vi "Json_New_Names_Test_Flo.vi"() -> ()   [LabVIEW 2014]
panel:
  out "JSON string":string="{\"label\":\"parms\",\"values\":[{\"chanDescs\":[{\"name\":\"HBCm_U30_01\",\"active\":1},{\"name\":\"HBCm_U30_02\",\"active\":1},{\"name\":\"HBCm_U30_03\",\"active\":1},{\"name\":\"HBCm_U30_04\",\"active\":1},{\"name\":\"HBCm_U30_05\",\"active\":1},{\"name\":\"HBCm_U30_06\",\"active\":1},{\"name\":\"HBCm_U30_07\",\"active\":1},{\"name\":\"HBCm_U30_08\",\"active\":1},{\"name\":\"HBCm_U30_09\",\"active\":1},{\"name\":\"HBCm_U30_10\",\"active\":1},{\"name\":\"HBCm_U30_11\",\"active\":1},{\"name\":\"HBCm_U30_12\",\"active\":1},{\"name\":\"HBCm_U30_13\",\"active\":1},{\"name\":\"HBCm_U30_14\",\"active\":1},{\"name\":\"HBCm_U30_15\",\"active\":1},{\"name\":\"HBCm_U30_16\",\"active\":1},{\"name\":\"HBCm_U30_17\",\"active\":1},{\"name\":\"HBCm_U30_18\",\"active\":1},{\"name\":\"HBCm_U30_19\",\"active\":1},{\"name\":\"HBCm_U30_20\",\"active\":1},{\"name\":\"HBCm_U30_21\",\"active\":1},{\"name\":\"HBCm_U30_22\",\"active\":1},{\"name\":\"HBCm_U30_23\",\"active\":1},{\"name\":\"HBCm_U30_24\",\"active\":1},{\"name\":\"HBCm_U30_25\",\"active\":1},{\"name\":\"HBCm_U30_26\",\"active\":1},{\"name\":\"HBCm_U30_27\",\"active\":1},{\"name\":\"HBCm_U30_28\",\"active\":1},{\"name\":\"HBCm_U30_29\",\"active\":1},{\"name\":\"HBCm_U30_30\",\"active\":1},{\"name\":\"HBCm_U30_31\",\"active\":1},{\"name\":\"HBCm_U30_32\",\"active\":1},{\"name\":\"HBCm_V21_01\",\"active\":1},{\"name\":\"HBCm_V21_02\",\"active\":1},{\"name\":\"HBCm_V21_03\",\"active\":1},{\"name\":\"HBCm_V21_04\",\"active\":1},{\"name\":\"HBCm_V21_05\",\"active\":1},{\"name\":\"HBCm_V21_06\",\"active\":1},{\"name\":\"HBCm_V21_07\",\"active\":1},{\"name\":\"HBCm_V21_08\",\"active\":1},{\"name\":\"HBCm_V21_09\",\"active\":1},{\"name\":\"HBCm_V21_10\",\"active\":1},{\"name\":\"HBCm_V21_11\",\"active\":1},{\"name\":\"HBCm_V21_12\",\"active\":1},{\"name\":\"HBCm_V21_13\",\"active\":1},{\"name\":\"HBCm_V21_14\",\"active\":1},{\"name\":\"HBCm_V21_15\",\"active\":1},{\"name\":\"HBCm_V21_16\",\"active\":1},{\"name\":\"HBCm_V21_17\",\"active\":1},{\"name\":\"HBCm_V21_18\",\"active\":1},{\"name\":\"HBCm_V21_19\",\"active\":1},{\"name\":\"HBCm_V21_20\",\"active\":1},{\"name\":\"HBCm_V21_21\",\"active\":1},{\"name\":\"HBCm_V21_22\",\"active\":1},{\"name\":\"HBCm_V21_23\",\"active\":1},{\"name\":\"HBCm_V21_24\",\"active\":1},{\"name\":\"HBCm_V21_25\",\"active\":1},{\"name\":\"HBCm_V21_26\",\"active\":1},{\"name\":\"HBCm_V21_27\",\"active\":1},{\"name\":\"HBCm_V21_28\",\"active\":1},{\"name\":\"HBCm_V21_29\",\"active\":1},{\"name\":\"HBCm_V21_30\",\"active\":1},{\"name\":\"HBCm_V21_31\",\"active\":1},{\"name\":\"HBCm_V21_32\",\"active\":1},{\"name\":\"HBCm_V21_33\",\"active\":1},{\"name\":\"HBCm_V21_34\",\"active\":1},{\"name\":\"HBCm_V21_35\",\"active\":1},{\"name\":\"HBCm_V21_36\",\"active\":1},{\"name\":\"HBCm_V21_37\",\"active\":1},{\"name\":\"HBCm_V21_38\",\"active\":1},{\"name\":\"HBCm_V21_39\",\"active\":1},{\"name\":\"HBCm_V21_40\",\"active\":1},{\"name\":\"VBCs_V21_01\",\"active\":1},{\"name\":\"VBCs_V21_02\",\"active\":1},{\"name\":\"VBCs_V21_03\",\"active\":1},{\"name\":\"VBCs_V21_04\",\"active\":1},{\"name\":\"VBCs_V21_05\",\"active\":1},{\"name\":\"VBCs_V21_06\",\"active\":1},{\"name\":\"VBCs_V21_08\",\"active\":1},{\"name\":\"VBCs_V21_09\",\"active\":0},{\"name\":\"VBCs_V21_01\",\"active\":1},{\"name\":\"VBCs_V21_02\",\"active\":1},{\"name\":\"VBCs_V21_03\",\"active\":1},{\"name\":\"VBCs_V21_04\",\"active\":1},{\"name\":\"VBCs_V21_05\",\"active\":1},{\"name\":\"VBCs_V21_06\",\"active\":1},{\"name\":\"VBCs_V21_07\",\"active\":1},{\"name\":\"VBCs_V21_08\",\"active\":1},{\"name\":\"VBCs_V21_09\",\"active\":1},{\"name\":\"VBCs_V21_09\",\"active\":1},{\"name\":\"VBCs_V21_10\",\"active\":1},{\"name\":\"VBCs_V21_11\",\"active\":1},{\"name\":\"VBCs_V21_12\",\"active\":1},{\"name\":\"VBCs_V21_13\",\"active\":1},{\"name\":\"VBCs_V21_14\",\"active\":1},{\"name\":\"VBCs_V21_15\",\"active\":1}]}],\"dimensions\":[1399090569999999999,-1]}"
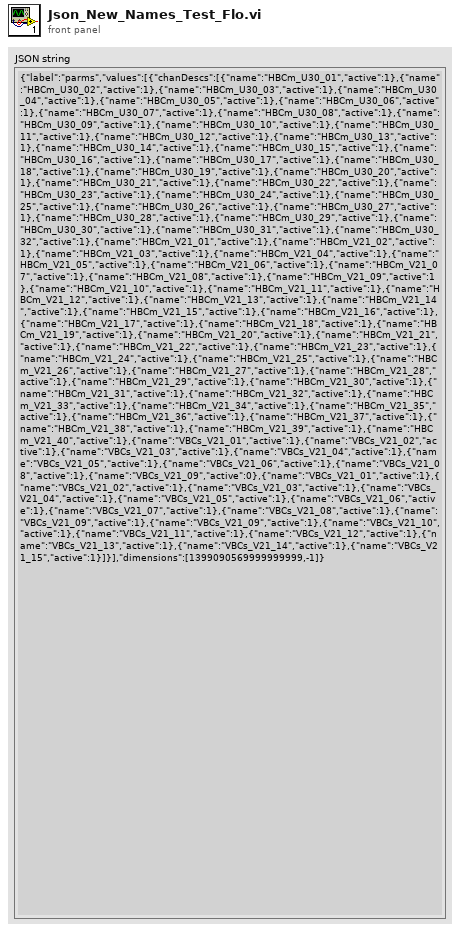
[diagram p1: front panel]
types:
  T1 = cluster{"chanDescs":cluster{"name":string, "active":i32}[]}[]
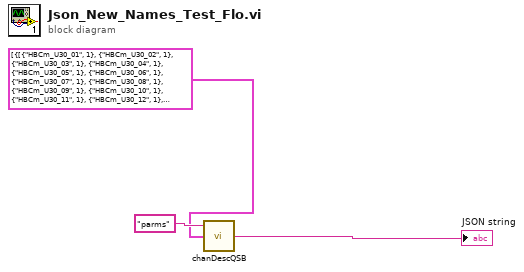
[diagram p0: block diagram]
diagram:
  n1 = call "chanDescQSB.vi"("values"=T1 [{"chanDescs"=[{"name"="HBCm_U30_01", "active"=1}, {"name"="HBCm_U30_02", "active"=1}, {"name"="HBCm_U30_03", "active"=1}, {"name"="HBCm_U30_04", "active"=1}, {"name"="HBCm_U30_05", "active"=1}, {"name"="HBCm_U30_06", "active"=1}, {"name"="HBCm_U30_07", "active"=1}, {"name"="HBCm_U30_08", "active"=1}, {"name"="HBCm_U30_09", "active"=1}, {"name"="HBCm_U30_10", "active"=1}, {"name"="HBCm_U30_11", "active"=1}, {"name"="HBCm_U30_12", "active"=1}, {"name"="HBCm_U30_13", "active"=1}, {"name"="HBCm_U30_14", "active"=1}, {"name"="HBCm_U30_15", "active"=1}, {"name"="HBCm_U30_16", "active"=1}, {"name"="HBCm_U30_17", "active"=1}, {"name"="HBCm_U30_18", "active"=1}, {"name"="HBCm_U30_19", "active"=1}, {"name"="HBCm_U30_20", "active"=1}, {"name"="HBCm_U30_21", "active"=1}, {"name"="HBCm_U30_22", "active"=1}, {"name"="HBCm_U30_23", "active"=1}, {"name"="HBCm_U30_24", "active"=1}, {"name"="HBCm_U30_25", "active"=1}, {"name"="HBCm_U30_26", "active"=1}, {"name"="HBCm_U30_27", "active"=1}, {"name"="HBCm_U30_28", "active"=1}, {"name"="HBCm_U30_29", "active"=1}, {"name"="HBCm_U30_30", "active"=1}, {"name"="HBCm_U30_31", "active"=1}, {"name"="HBCm_U30_32", "active"=1}, {"name"="VBCm_V21_01", "active"=1}, {"name"="VBCm_V21_02", "active"=1}, {"name"="VBCm_V21_03", "active"=1}, {"name"="VBCm_V21_04", "active"=1}, {"name"="VBCm_V21_05", "active"=1}, {"name"="VBCm_V21_06", "active"=1}, {"name"="VBCm_V21_07", "active"=1}, {"name"="VBCm_V21_08", "active"=1}, {"name"="VBCm_V21_09", "active"=1}, {"name"="VBCm_V21_10", "active"=1}, {"name"="VBCm_V21_11", "active"=1}, {"name"="VBCm_V21_12", "active"=1}, {"name"="VBCm_V21_13", "active"=1}, {"name"="VBCm_V21_14", "active"=1}, {"name"="VBCm_V21_15", "active"=1}, {"name"="VBCm_V21_16", "active"=1}, {"name"="VBCm_V21_17", "active"=1}, {"name"="VBCm_V21_18", "active"=1}, {"name"="VBCm_V21_19", "active"=1}, {"name"="VBCm_V21_20", "active"=1}, {"name"="VBCm_V21_21", "active"=1}, {"name"="VBCm_V21_22", "active"=1}, {"name"="VBCm_V21_23", "active"=1}, {"name"="VBCm_V21_24", "active"=1}, {"name"="VBCm_V21_25", "active"=1}, {"name"="VBCm_V21_26", "active"=1}, {"name"="VBCm_V21_27", "active"=1}, {"name"="VBCm_V21_28", "active"=1}, {"name"="VBCm_V21_29", "active"=1}, {"name"="VBCm_V21_30", "active"=1}, {"name"="VBCm_V21_31", "active"=1}, {"name"="VBCm_V21_32", "active"=1}, {"name"="VBCm_V21_33", "active"=1}, {"name"="VBCm_V21_34", "active"=1}, {"name"="VBCm_V21_35", "active"=1}, {"name"="VBCm_V21_36", "active"=1}, {"name"="VBCm_V21_37", "active"=1}, {"name"="VBCm_V21_38", "active"=1}, {"name"="VBCm_V21_39", "active"=1}, {"name"="VBCm_V21_40", "active"=1}, {"name"="VBCs_V21_01", "active"=1}, {"name"="VBCs_V21_02", "active"=1}, {"name"="VBCs_V21_03", "active"=1}, {"name"="VBCs_V21_04", "active"=1}, {"name"="VBCs_V21_05", "active"=1}, {"name"="VBCs_V21_06", "active"=1}, {"name"="VBCs_V21_07", "active"=1}, {"name"="VBCs_V21_08", "active"=1}, {"name"="HBCs_U30_01", "active"=1}, {"name"="HBCs_U30_02", "active"=1}, {"name"="HBCs_U30_03", "active"=1}, {"name"="HBCs_U30_04", "active"=1}, {"name"="HBCs_U30_05", "active"=1}, {"name"="HBCs_U30_06", "active"=1}, {"name"="HBCs_U30_07", "active"=1}, {"name"="HBCs_U30_08", "active"=1}, {"name"="HBCs_U30_09", "active"=1}, {"name"="HBCs_U30_10", "active"=1}, {"name"="HBCs_U30_11", "active"=1}, {"name"="HBCs_U30_12", "active"=1}, {"name"="HBCs_U30_13", "active"=1}, {"name"="HBCs_U30_14", "active"=1}, {"name"="HBCs_U30_15", "active"=1}, {"name"="HBCs_U30_16", "active"=1}, {"name"="Bolo96", "active"=1}, {"name"="Bolo97", "active"=1}, {"name"="Bolo98", "active"=1}, {"name"="Bolo99", "active"=1}, {"name"="Bolo100", "active"=1}]}], "label"="parms") -> ("JSON string"=→"JSON string":string)  [unwired: 1 in]
